vi "FetchImageList (SubVI).vi"(8 "error in (no error)":errorcluster, 10 "Naming Convention":string="*.png", 11 "Images Directory":path=path "E:/XYZstage+Camera_CollectedImages/12-16-2016/noStaveMount/toolingpins_images") -> (0 "error out":errorcluster, 2 "List of Image Names":string[](array[string]), 3 "List of Image Paths":path[](array[path]), 5 "Filenames Array":string[](array[string]))   [LabVIEW 2016]
uses:
  <vilib>/regexp/Match Regular Expression.xnode
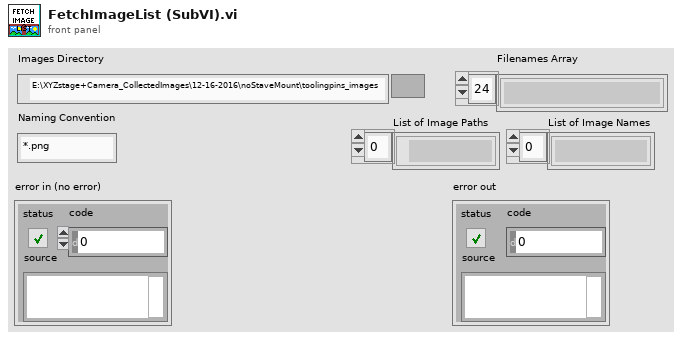
[diagram p1: front panel]
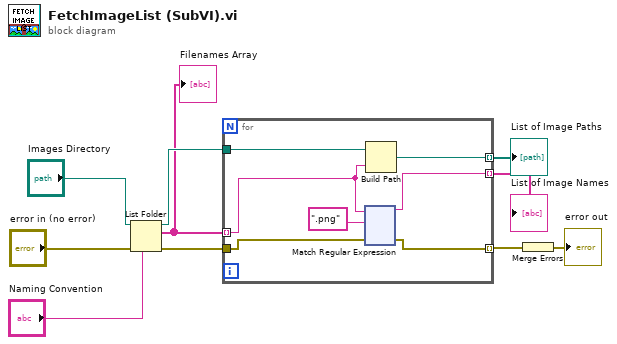
[diagram p0: block diagram]
diagram:
  n1 = List Folder(path="Images Directory", pattern="Naming Convention", error in="error in (no error)") -> (path out=w7:path, filenames=w3:string[], error out=w8:errorcluster)  [unwired: 1 in, 1 out]
  "Filenames Array" <- w3
  n2 = for {
    tunnel: w3 -> [w16] mode=indexing
    tunnel: w7 -> [w17]
    tunnel: w8 -> [w14]
    tunnel: [w13] -> w9 mode=indexing
    tunnel: [w12] -> w1 mode=indexing
    tunnel: [w11] -> w2 mode=indexing
    n3 = xnode "Match Regular Expression"("input string"=w16, "regular expression"=".png", "error in"=w14) -> ("before match"=w12:string, "error out"=w13:errorcluster)  [unwired: 3 in, 3 out]
    n4 = Build Path(base path=w17, name or relative path=w16) -> (appended path=w11:path)
  }
  "List of Image Paths" <- w2
  "List of Image Names" <- w1
  n5 = Merge Errors(w9) -> (→"error out":errorcluster)
